vi "SEA_9811_get_VS_conf.vi"(8 "error in (no error)":errorcluster, 11 "Device Reference in":T1 format="%.0x") -> (0 "error out":errorcluster, 1 "Transmit Channels Ref":T1 format="%.0x", 2 "SEA9811_conf_cluster":T2={"FPGA resource name"="RIO0", "Rx ch conf (0..7)"=[{"Rx Channel Number (0..7)"=0, "Rx Label Filter"={"Label 00"=0, "Label 01"=0, "Label 02"=0, "Label 03"=0, "Label 04"=0, "Label 05"=0, "Label 06"=0, "Label 07"=0, "Label 08"=0, "Label 09"=0, "Label 10"=0, "Label 11"=0, "Label 12"=0, "Label 13"=0, "Label 14"=0, "Label 15"=0}, "Receiver Control Register (RCR)"={"RCR0: Data rate = ARINC 429 High-Speed (0) or Low-Speed (1)"=FALSE, "RCR1: not used"=FALSE, "RCR2: Label recognition for this channel enabled (1) or disabled (0)"=FALSE, "RCR3: Receiver channel disabled (1) or enabled (0)"=FALSE, "RCR4: Odd parity check for this channel enabled (1) or disabled (0"=FALSE, "RCR5: Receiver normal operation (1) or loopback mode (0)"=TRUE, "RCR6: Receiver Decoder disabled (0) or enabled (1) \n-> ARINC bits 10 and 9 must match RCR7 and RCR8"=FALSE, "RCR7: If receiver decoder is enabled (RCR6=1), \nthe ARINC bit 10 must match this bit"=FALSE, "RCR8: If receiver decoder is enabled (RCR6=1), \nthe ARINC bit 9 must match this bit"=FALSE, "RCR9: Label bit order for this channel non-reversed (1) \nor reversed (0)"=FALSE, "RCR10: not used"=FALSE, "RCR11: not used"=FALSE, "RCR12: not used"=FALSE, "RCR13: not used"=FALSE, "RCR14: not used"=FALSE, "RCR15: not used"=FALSE}}], "Transmitter Control Register (TCR)"={"TCR0: not used"=FALSE, "TCR1: not used"=FALSE, "TCR2: not used"=FALSE, "TCR3: Transmitter Parity Bit Enable: 32nd bit is parity (1) or data (0)"=FALSE, "TCR4: not used"=FALSE, "TCR5: not used"=FALSE, "TCR6: not used"=FALSE, "TCR7: not used"=FALSE, "TCR8: not used"=FALSE, "TCR9: Transmitter Parity Select: odd parity (0) or even parity (1)"=FALSE, "TCR10: Transmitter Data Rate: ARINC 429 high-speed (0) or low-speed (1)"=FALSE, "TCR11: ARINC Label Bit Order: label bit order reversed (0) or not reversed (1)"=FALSE, "TCR12: Disable Line Driver: normal operation (0) or transmitter disabled (1)"=FALSE, "TCR13: Tansmit whenever data is available in FIFO (1) or only start by instruction \"Enable Transmission\" (0)"=TRUE, "TCR14: not used"=FALSE, "TCR15: not used"=FALSE}, "Bitfile Path"=path ""}, 3 "Device Reference out":T1 format="%.0x", 5 "NIVS FPGA Personality?":bool)   [LabVIEW 2015]
uses:
  <vilib>/NI Veristand/Custom Device API/Custom Device Item Ref.ctl
  Typdefs/SEA9811_RT_conf_cluster.ctl
  <vilib>/userdefined/High Color/nirio_resource_hc.ctl
  FPGA/SEA-9811_ReceiverAndTransmitter/SubVIs/SEA-9811_ReceiverAndTransmitter_RCR.ctl
  FPGA/SEA-9811_ReceiverAndTransmitter/SubVIs/SEA-9811_ReceiverAndTransmitter_TCR.ctl
  Shared/Controls and Global/Global.vi
  <vilib>/NI Veristand/Custom Device API/Get Item Property (Variant).vi
  <vilib>/NI Veristand/Custom Device API/Get Item Property (String).vi
  <vilib>/NI Veristand/Custom Device API/Get Item Property (Boolean).vi
  <vilib>/NI Veristand/Custom Device API/Get Item Property (Path).vi
  <vilib>/NI Veristand/Custom Device Tools/Custom Device Utility Library/NI VeriStand - Search for Item by Name.vi
  <vilib>/NI VeriStand/Custom Device API/Custom Device API.lvlib
  Shared/ARINC 429 Shared.lvlib
  <vilib>/NI VeriStand/Custom Device Tools/Custom Device Utility Library/Custom Device Utility Library.lvlib
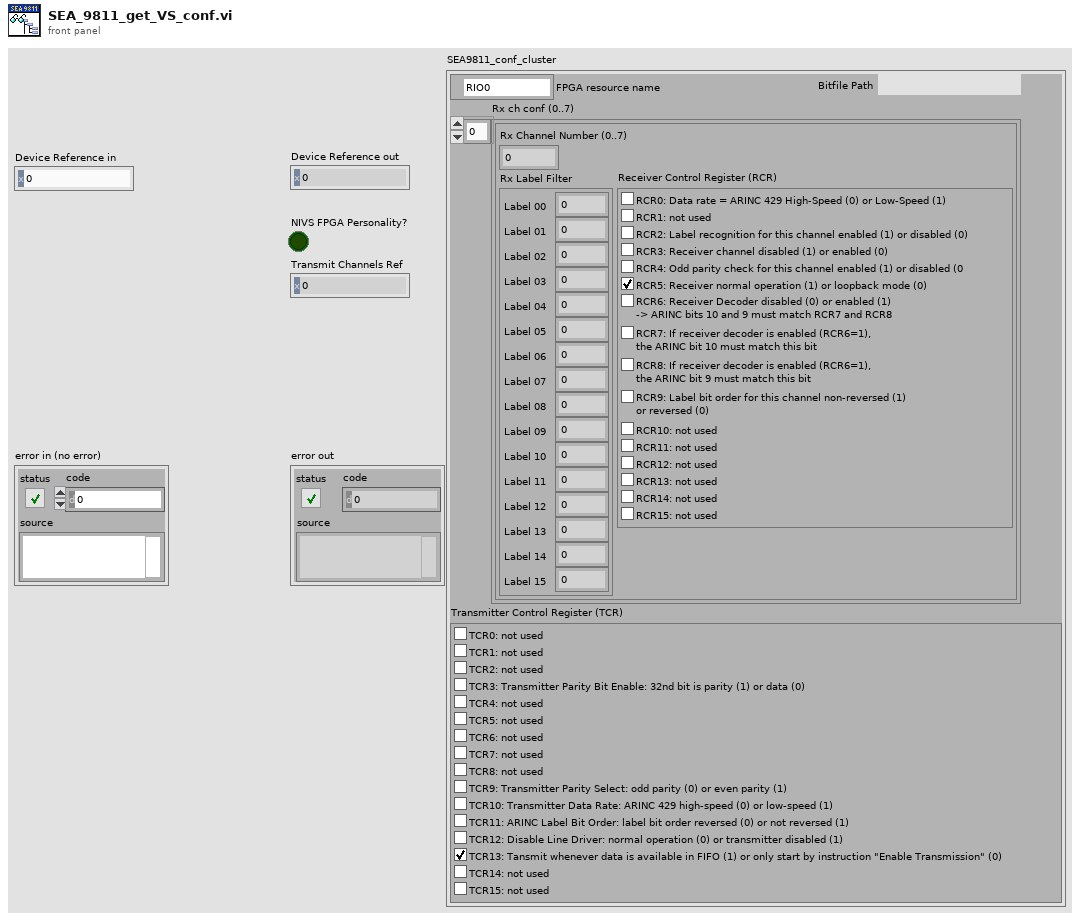
[diagram p1: front panel]
types:
  T1 = typedef "Custom Device API.lvlib/Custom Device Item Ref.ctl" = u64
  T2 = typedef "SEA9811_RT_conf_cluster.ctl" = cluster{"FPGA resource name":T3, "Rx ch conf (0..7)":cluster{"Rx Channel Number (0..7)":u8, "Rx Label Filter":cluster{"Label 00":u8, "Label 01":u8, "Label 02":u8, "Label 03":u8, "Label 04":u8, "Label 05":u8, "Label 06":u8, "Label 07":u8, "Label 08":u8, "Label 09":u8, "Label 10":u8, "Label 11":u8, "Label 12":u8, "Label 13":u8, "Label 14":u8, "Label 15":u8}, "Receiver Control Register (RCR)":T4}[], "Transmitter Control Register (TCR)":T5, "Bitfile Path":path}
  T3 = typedef "nirio_resource_hc.ctl" = tag
  T4 = typedef "SEA-9811_ReceiverAndTransmitter_RCR.ctl" = cluster{"RCR0: Data rate = ARINC 429 High-Speed (0) or Low-Speed (1)":bool, "RCR1: not used":bool, "RCR2: Label recognition for this channel enabled (1) or disabled (0)":bool, "RCR3: Receiver channel disabled (1) or enabled (0)":bool, "RCR4: Odd parity check for this channel enabled (1) or disabled (0":bool, "RCR5: Receiver normal operation (1) or loopback mode (0)":bool, "RCR6: Receiver Decoder disabled (0) or enabled (1) \n-> ARINC bits 10 and 9 must match RCR7 and RCR8":bool, "RCR7: If receiver decoder is enabled (RCR6=1), \nthe ARINC bit 10 must match this bit":bool, "RCR8: If receiver decoder is enabled (RCR6=1), \nthe ARINC bit 9 must match this bit":bool, "RCR9: Label bit order for this channel non-reversed (1) \nor reversed (0)":bool, "RCR10: not used":bool, "RCR11: not used":bool, "RCR12: not used":bool, "RCR13: not used":bool, "RCR14: not used":bool, "RCR15: not used":bool}
  T5 = typedef "SEA-9811_ReceiverAndTransmitter_TCR.ctl" = cluster{"TCR0: not used":bool, "TCR1: not used":bool, "TCR2: not used":bool, "TCR3: Transmitter Parity Bit Enable: 32nd bit is parity (1) or data (0)":bool, "TCR4: not used":bool, "TCR5: not used":bool, "TCR6: not used":bool, "TCR7: not used":bool, "TCR8: not used":bool, "TCR9: Transmitter Parity Select: odd parity (0) or even parity (1)":bool, "TCR10: Transmitter Data Rate: ARINC 429 high-speed (0) or low-speed (1)":bool, "TCR11: ARINC Label Bit Order: label bit order reversed (0) or not reversed (1)":bool, "TCR12: Disable Line Driver: normal operation (0) or transmitter disabled (1)":bool, "TCR13: Tansmit whenever data is available in FIFO (1) or only start by instruction \"Enable Transmission\" (0)":bool, "TCR14: not used":bool, "TCR15: not used":bool}
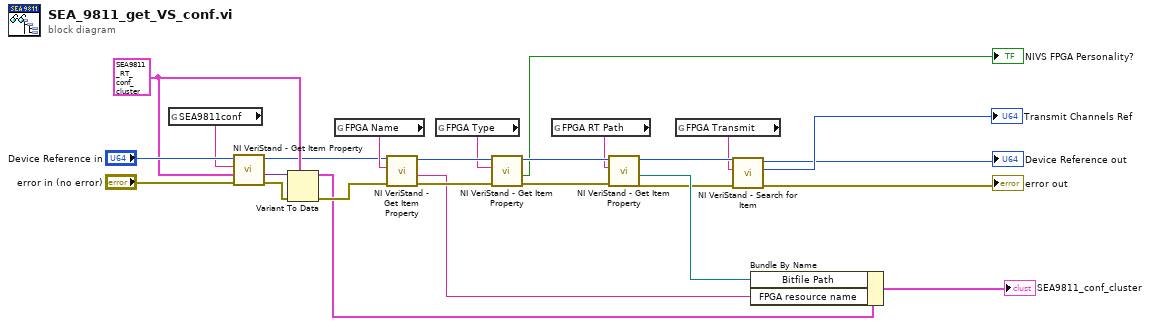
[diagram p0: block diagram]
diagram:
  w21 = T2 {"FPGA resource name"="RIO0", "Rx ch conf (0..7)"=[], "Transmitter Control Register (TCR)"={"TCR0: not used"=FALSE, "TCR1: not used"=FALSE, "TCR2: not used"=FALSE, "TCR3: Transmitter Parity Bit Enable: 32nd bit is parity (1) or data (0)"=FALSE, "TCR4: not used"=FALSE, "TCR5: not used"=FALSE, "TCR6: not used"=FALSE, "TCR7: not used"=FALSE, "TCR8: not used"=FALSE, "TCR9: Transmitter Parity Select: odd parity (0) or even parity (1)"=FALSE, "TCR10: Transmitter Data Rate: ARINC 429 high-speed (0) or low-speed (1)"=FALSE, "TCR11: ARINC Label Bit Order: label bit order reversed (0) or not reversed (1)"=FALSE, "TCR12: Disable Line Driver: normal operation (0) or transmitter disabled (1)"=FALSE, "TCR13: Tansmit whenever data is available in FIFO (1) or only start by instruction \"Enable Transmission\" (0)"=TRUE, "TCR14: not used"=FALSE, "TCR15: not used"=FALSE}, "Bitfile Path"=path ""} ("SEA9811_conf_cluster")
  n1 = global read "Global.vi" "SEA9811conf"() -> (w25:string)
  n2 = call-poly <vilib>:"NI VeriStand - Get Item Property.vi"("error in (no error)"="error in (no error)", "Default Value"=w21, "Property Name"=w25, "Item Ref in"="Device Reference in") -> ("error out"=w22:errorcluster, "Value"=w23:variant, "Item Ref out"=w13:T1)  [unwired: 4 in, 1 out]
  n3 = Variant To Data(error in=w22, type=w21, Variant=w23) -> (data=w11:T2, error out=w12:errorcluster)
  n4 = global read "Global.vi" "FPGA Name"() -> (w16:string)
  n5 = call-poly <vilib>:"NI VeriStand - Get Item Property.vi"("error in (no error)"=w12, "Property Name"=w16, "Item Ref in"=w13) -> ("error out"=w20:errorcluster, "Value"=w9:string, "Item Ref out"=w19:T1)  [unwired: 5 in, 1 out]
  n6 = global read "Global.vi" "FPGA Type"() -> (w15:string)
  n7 = call-poly <vilib>:"NI VeriStand - Get Item Property.vi"("error in (no error)"=w20, "Property Name"=w15, "Item Ref in"=w19) -> ("error out"=w17:errorcluster, "Value"=→"NIVS FPGA Personality?":bool, "Item Ref out"=w18:T1)  [unwired: 5 in, 1 out]
  n8 = global read "Global.vi" "FPGA RT Path"() -> (w14:string)
  n9 = call-poly <vilib>:"NI VeriStand - Get Item Property.vi"("error in (no error)"=w17, "Property Name"=w14, "Item Ref in"=w18) -> ("error out"=w5:errorcluster, "Value"=w8:path, "Item Ref out"=w6:T1)  [unwired: 5 in, 1 out]
  n10 = global read "Global.vi" "FPGA Transmit"() -> (w4:string)
  n11 = call-poly <vilib>:"NI VeriStand - Search for Item.vi"("error in"=w5, "Item Name"=w4, "Section Ref in"=w6) -> ("error out"=→"error out":errorcluster, "Item Ref"=→"Transmit Channels Ref":T1, "Section Ref out"=→"Device Reference out":T1)  [unwired: 5 in, 1 out]
  n12 = Bundle By Name(cluster=w11, "Bitfile Path"=w8, "FPGA resource name"=w9) -> (→"SEA9811_conf_cluster":T2)
